vi "Map_Init.vi"(0 "object in":refnum<class "Map.lvclass">, 5 "error in (no error)":errorcluster) -> (14 "object out":refnum<class "Map.lvclass">, 19 "error out":errorcluster)   [LabVIEW 2015, in "Map.lvclass"]
doc: "Creates a 10x10 map."
uses:
  Map.lvclass
  TypDefs/ShipType.ctl
  TypDefs/GameType.ctl
  TypDefs/Coordinates.ctl
  Map.lvclass/Map.ctl
  Battleship_class/Battleship.lvclass
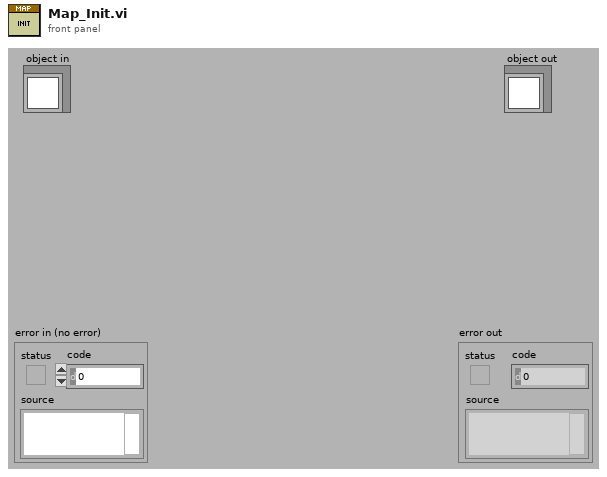
[diagram p1: front panel]
types:
  T1 = typedef "Coordinates.ctl" = cluster{"X":i32, "Y":i32}
  T2 = typedef "GameType.ctl" = enum16{"Classic", "Modern"}
  T3 = typedef "ShipType.ctl" = enum16{"Carrier", "Destroyer", "Submarine", "Frigate", "Scout"}
  T4 = cluster{"Sea":u32, "Ship":u32, "Hit":u32, "Miss":u32}
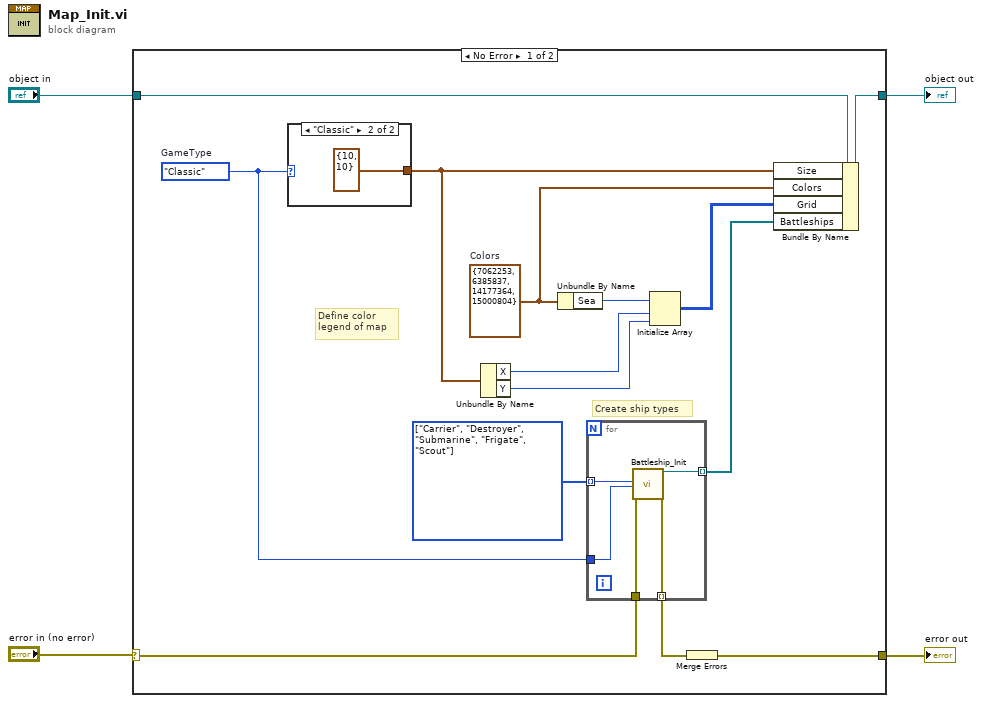
[diagram p0: block diagram]
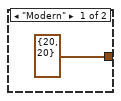
[diagram p2: hidden frame]
diagram:
  n1 = case shown="No Error" "error in (no error)" {
    selector: "error in (no error)" -> [w12 w26]
    tunnel: "object in" -> [w18 w27]
    tunnel: [w17 w27] -> w3
    tunnel: [w10 w26] -> w1
    frame No Error {
      w5 = GameType."Classic"  # GameType
      w14 = T3[] [enum."Carrier", enum."Destroyer", enum."Submarine", enum."Frigate", enum."Scout"] items=["Carrier", "Destroyer", "Submarine", "Frigate", "Scout"]
      w7 = T4 {"Sea"=7062253, "Ship"=6385837, "Hit"=14177364, "Miss"=15000804}  # Colors
      # "Create ship types"
      # "Define color\nlegend of map"
      n2 = case shown="\"Classic\"" w5 {
        tunnel: [T1 {"X"=20, "Y"=20} ("Size") T1 {"X"=10, "Y"=10} ("Size")] -> w9
        frame "Modern" {
        }
        frame "Classic" {
        }
      }
      n3 = Unbundle By Name(w9) -> ("X"=w16:i32, "Y"=w15:i32)
      n4 = Unbundle By Name(w7) -> ("Sea"=w8:u32)
      n5 = for {
        tunnel: w14 -> [w25] mode=indexing
        tunnel: [w24] -> w13 mode=indexing
        tunnel: w12 -> [w23]
        tunnel: [w22] -> w11 mode=indexing
        tunnel: w5 -> [w21]
        n6 = call "Battleship_Init.vi"("ShipType"=w25, "GameType"=w21, "error in (no error)"=w23) -> ("object out"=w24:refnum<class "Battleship.lvclass">, "error out"=w22:errorcluster)  [unwired: 15 in]
      }
      n7 = Initialize Array(w8, w16, w15) -> (w6:u32[][])
      n8 = Merge Errors(w11) -> (w10:errorcluster)
      n9 = Bundle By Name(cluster=w18, "Size"=w9, "Colors"=w7, "Grid"=w6, "Battleships"=w13) -> (w17:refnum<class "Map.lvclass">)
    }
    frame Error {
    }
  }
  "object out" <- w3
  "error out" <- w1
